vi "Check Output State.vi"(8 "error in (no error)":errorcluster, 11 "VISA resource name":refnum<visa-resource-name>) -> (0 "error out":errorcluster, 2 "Output":bool, 3 "VISA resource name out":refnum<visa-resource-name>)   [LabVIEW 2020, in "MagnaDC.lvlib"]
doc: "Configures output voltage level, channel, and enables or disables the output of the power supply."
uses:
  MagnaDC.lvlib
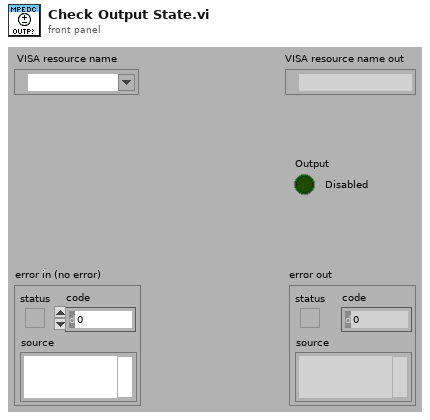
[diagram p1: front panel]
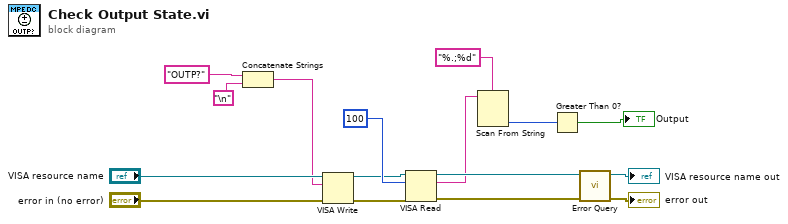
[diagram p0: block diagram]
diagram:
  n1 = Concatenate Strings("OUTP?", "\n") -> (w11:string)
  n2 = VISA Write(VISA resource name="VISA resource name", write buffer=w11, error in (no error)="error in (no error)") -> (VISA resource name out=w8:refnum<visa-resource-name>, error out=w7:errorcluster)  [unwired: 1 out]
  n3 = VISA Read(VISA resource name=w8, byte count=u32 100, error in (no error)=w7) -> (VISA resource name out=w6:refnum<visa-resource-name>, read buffer=w4:string, error out=w5:errorcluster)  [unwired: 1 out]
  n4 = Scan From String(format string="%.;%d", input string=w4) -> (output 1=w2:i32)  [unwired: 3 in, 3 out]
  n5 = Greater Than 0?(x=w2) -> (x > 0?=→"Output":bool)
  n6 = call "Error Query.vi"("error in (no error)"=w5, "VISA resource name"=w6) -> ("error out"=→"error out":errorcluster, "VISA resource name out"=→"VISA resource name out":refnum<visa-resource-name>)  [unwired: 6 in, 2 out]
